vi "Write Shared Key.vi"(8 "error in (no error)":errorcluster, 10 "Shared Key":string, 11 "Attribute.Owner in":refnum<class "Attribute.Owner.lvclass">) -> (0 "error out":errorcluster, 3 "Attribute.Owner out":refnum<class "Attribute.Owner.lvclass">)   [LabVIEW 2013, in "Attribute.Owner.lvclass"]
uses:
  Attribute.Owner.lvclass
  Attribute.Owner.lvclass/Attribute.Owner.ctl
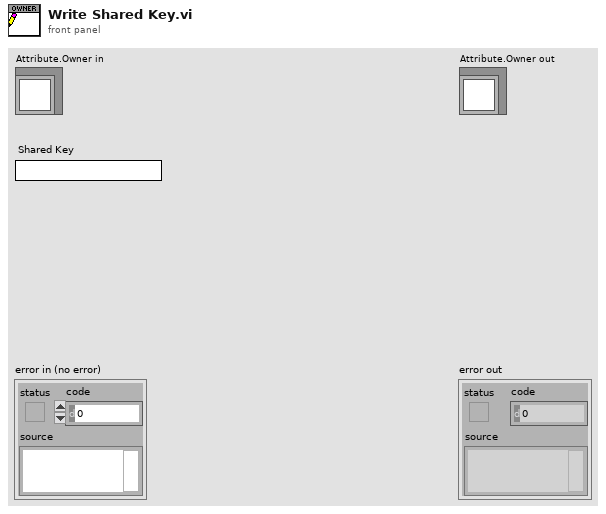
[diagram p1: front panel]
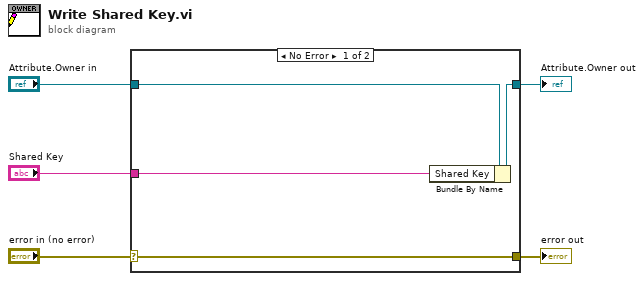
[diagram p0: block diagram]
diagram:
  n1 = case shown="No Error" "error in (no error)" {
    selector: "error in (no error)" -> [w9 w10]
    tunnel: [w9 w10] -> w4
    tunnel: [w7 w11] -> w2
    tunnel: "Attribute.Owner in" -> [w8 w11]
    tunnel: "Shared Key" -> [w6 _]
    frame No Error {
      n2 = Bundle By Name(cluster=w8, "Shared Key"=w6) -> (w7:refnum<class "Attribute.Owner.lvclass">)
    }
    frame Error {
    }
  }
  "error out" <- w4
  "Attribute.Owner out" <- w2
